vi "Convert Degrees to Radians.vi"(1 "Deg":dbl format="%.2f") -> (0 "rad":dbl format="%.2f")   [LabVIEW 2015]
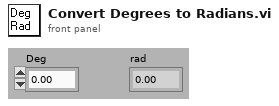
[diagram p1: front panel]
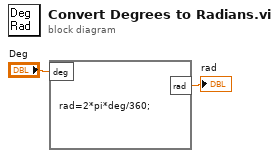
[diagram p0: block diagram]
diagram:
  n1 = formula code="rad=2*pi*deg/360;"("deg"="Deg") -> ("rad"=→"rad":dbl)
